vi "Test structure-Event.vi"   [LabVIEW 2026]
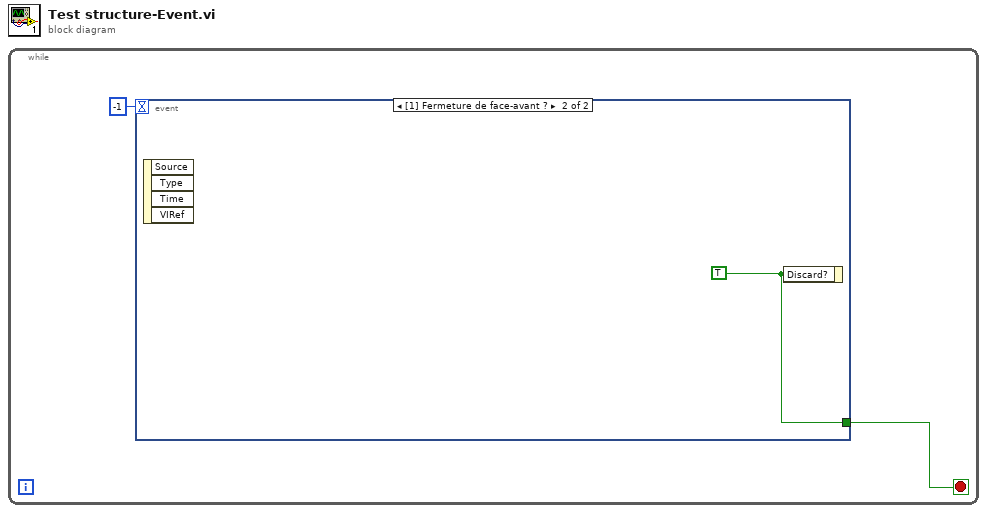
[diagram p0: block diagram]
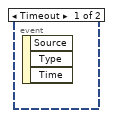
[diagram p2: hidden frame]
diagram:
  n1 = while {
    stop <- w1 stop-if-true
    n2 = event shown="[1] Fermeture de face-avant ?" {
      selector: _ -> [_ _]
      dyn-events: _ -> [_ _]
      timeout: -1 -> [_ _]
      tunnel: [_ w3] -> w1
      event Timeout {
        n3 = event-data() -> ()  [unwired: 1 in, 3 out]
      }
      event Panel Close? {
        w3 = TRUE ("Rejeter ?")
        n4 = event-data() -> ()  [unwired: 1 in, 4 out]
        n5 = event-data("Discard?"=w3) -> ()  [unwired: 1 in, 1 out]
      }
    }
  }
